vi "Generador de 15.vi"(8 "Semilla 2":u16, 9 "Semilla 1":u16, 11 "Modo":enum16{"Insertar Semillas", "Generar"}(ring)) -> (3 "Recorrdo":u16 format="%b")   [LabVIEW 2023]
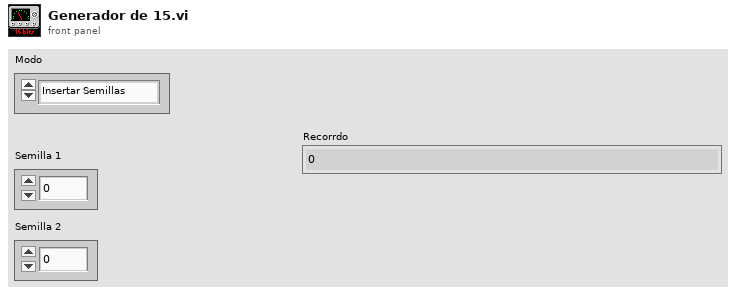
[diagram p1: front panel]
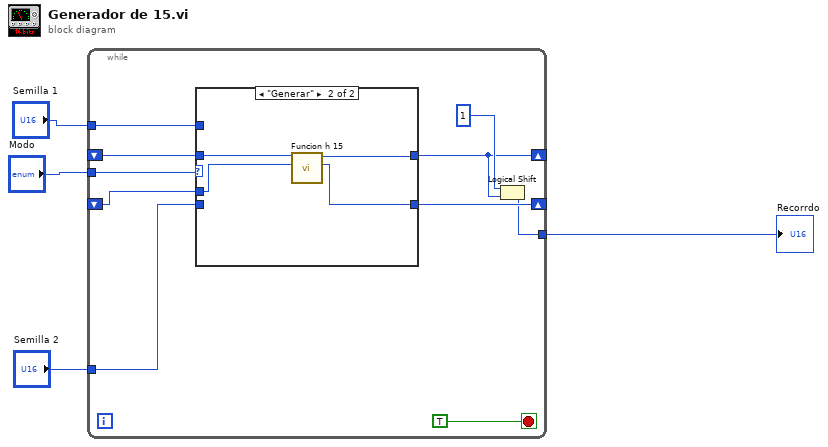
[diagram p0: block diagram]
diagram:
  n1 = while {
    tunnel: "Modo" -> [w13]
    shift-right: [w5] -> _
    shift-left: _ -> [w9]
    shift-right: [w12] -> _
    shift-left: _ -> [w8]
    tunnel: "Semilla 1" -> [w11]
    tunnel: "Semilla 2" -> [w10]
    tunnel: [w7] -> w1
    stop <- TRUE stop-if-true
    n2 = case shown="\"Generar\"" w13 {
      tunnel: [w16 w17] -> w5
      tunnel: [w15 w18] -> w12
      tunnel: w11 -> [w16 _]
      tunnel: w10 -> [w15 _]
      tunnel: w9 -> [_ w20]
      tunnel: w8 -> [_ w19]
      frame "Insertar Semillas", Default {
      }
      frame "Generar" {
        n3 = call "Funcion h 15.vi"("y"=w19, "x"=w20) -> ("y(t+1)"=w18:u16, "x(t+1)"=w17:u16)  [unwired: 8 in]
      }
    }
    n4 = Logical Shift(y=u16 1 ("x"), x=w5) -> (x << y=w7:u16)
  }
  "Recorrdo" <- w1
